vi "New Value Change Trigger.vi"(8 "error in (no error)":errorcluster, 11 "Deadband":dbl) -> (0 "error out":errorcluster, 3 "Value Change Trigger out":refnum<class "Value Change Trigger.lvclass">)   [LabVIEW 2015, in "Waveform Data Logger Engine.lvlib" / "Value Change Trigger.lvclass"]
uses:
  Value Change Trigger.lvclass
  Value Change Trigger.lvclass/Value Change Trigger.ctl
  Trigger/Trigger Type.ctl
  Trigger/Trigger.lvclass/Trigger.ctl
  Trigger/Write Trigger Type.vi
  Trigger/Trigger.lvclass
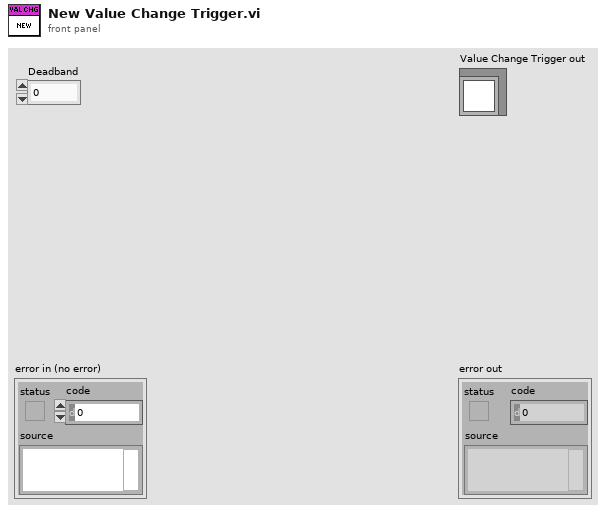
[diagram p1: front panel]
types:
  T1 = typedef "Waveform Data Logger Engine.lvlib/Trigger.lvclass/Trigger Type.ctl" = enum16{"Default", "Digital Edge", "Analog Edge", "In Range", "Value Change", "Boolean Evaluation"}
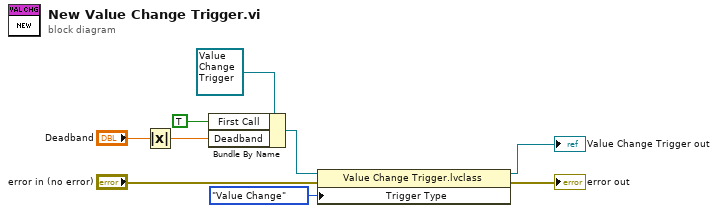
[diagram p0: block diagram]
diagram:
  n1 = Absolute Value(x="Deadband") -> (abs(x)=w6:dbl)
  n2 = Bundle By Name(cluster=refnum<class "Value Change Trigger.lvclass"> refnum ("Value Change Trigger in"), "First Call"=TRUE, "Deadband"=w6) -> (w5:refnum<class "Value Change Trigger.lvclass">)
  n3 = property class="Value Change Trigger.lvclass"(reference=w5, error in="error in (no error)", "Trigger Type"=Trigger_Type."Value Change") -> (reference out=→"Value Change Trigger out":refnum<class "Value Change Trigger.lvclass">, error out=→"error out":errorcluster)
